vi "read_position.vi"(0 "handle in":i32, 11 "error in (no error)":errorcluster) -> (4 "handle out":i32, 6 "x":dbl, 8 "y":dbl, 10 "z":dbl, 15 "error out":errorcluster)   [LabVIEW 2019]
uses:
  controller/SubVIs_nanostage/Madlib.dll
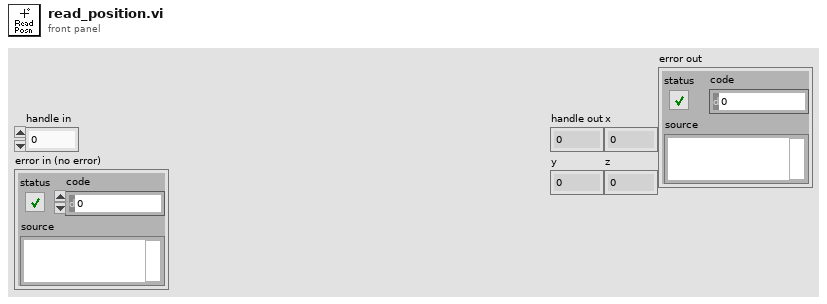
[diagram p1: front panel]
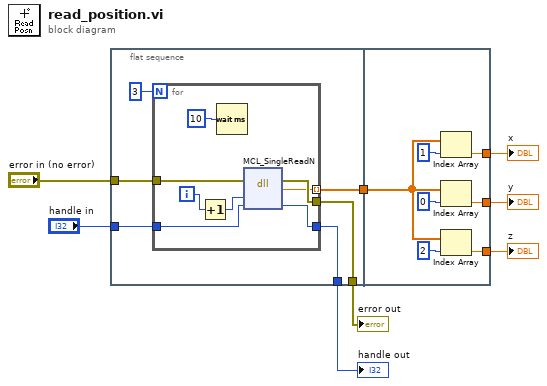
[diagram p0: block diagram]
diagram:
  n1 = flat-sequence {
    tunnel: [w13] -> w8
    tunnel: "handle in" -> [w12]
    tunnel: "error in (no error)" -> [w11]
    tunnel: [w10] -> w5
    tunnel: [w9] -> w1
    tunnel: w8 -> [w26]
    tunnel: [w25] -> w4
    tunnel: [w24] -> w3
    tunnel: [w23] -> w2
    frame #0 {
      n2 = for {
        N: 3 -> [_]
        tunnel: [w19] -> w9
        tunnel: [w20] -> w10
        tunnel: [w18] -> w13 mode=indexing
        tunnel: w12 -> [w17]
        tunnel: w11 -> [w16]
        i -> [w15]
        n3 = Increment(x=w15) -> (x+1=w22:i32)
        n4 = Wait (ms)(milliseconds to wait=u32 10) -> ()  [unwired: 1 out]
        n5 = dll-call lib="C:/Users/admin/Desktop/controller/SubVIs_nanostage/MADLib.dll" fn="MCL_SingleReadN" label="Read Posn"(error in=w16, "axis"=w22, "handle"=w17) -> (error out=w19:errorcluster, "position"=w18:dbl, "handle"=w20:i32)  [unwired: 3 in, 1 out]
      }
    }
    frame #1 {
      n6 = Index Array(array=w26, index=1) -> (element=w25:dbl)
      n7 = Index Array(array=w26, index=0) -> (element=w24:dbl)
      n8 = Index Array(array=w26, index=2) -> (element=w23:dbl)
    }
  }
  "handle out" <- w5
  "x" <- w4
  "y" <- w3
  "z" <- w2
  "error out" <- w1
